vi "Init State Machine.vi"(8 "error in (no error)":errorcluster, 11 "Channel in":refnum<class "Channel.lvclass">) -> (0 "error out":errorcluster, 3 "Channel out":refnum<class "Channel.lvclass">)   [LabVIEW 2018, in "Channel.lvclass"]
doc: "Initialize state machine"
uses:
  Channel.lvclass
  Channel.lvclass/Channel.ctl
  State Machine/CCS_State Machine.lvclass
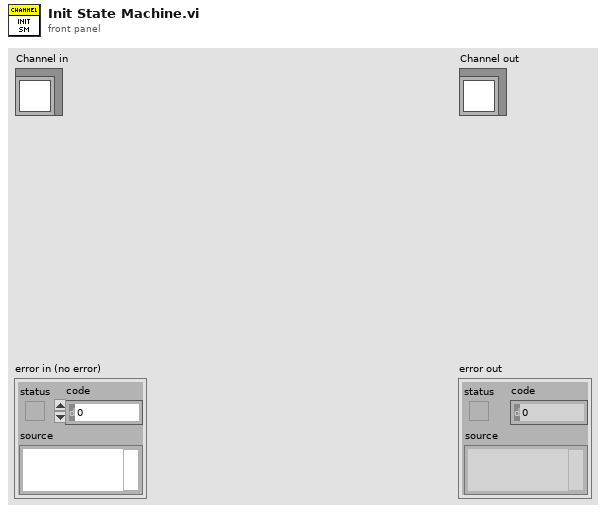
[diagram p1: front panel]
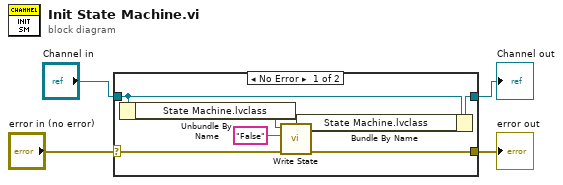
[diagram p0: block diagram]
diagram:
  n1 = case shown="No Error" "error in (no error)" {
    selector: "error in (no error)" -> [w10 w13]
    tunnel: [w11 w13] -> w3
    tunnel: [w8 w12] -> w1
    tunnel: "Channel in" -> [w9 w12]
    frame No Error {
      n2 = Unbundle By Name(w9) -> ("State Machine.lvclass"=w6:refnum<class "CCS_State Machine.lvclass">)
      n3 = call-dynamic "Write State.vi"("error in (no error)"=w10, "State"="False", "State Machine in"=w6) -> ("error out"=w11:errorcluster, "State Machine out"=w5:refnum<class "CCS_State Machine.lvclass">)  [unwired: 7 in]
      n4 = Bundle By Name(cluster=w9, "State Machine.lvclass"=w5) -> (w8:refnum<class "Channel.lvclass">)
    }
    frame Error {
    }
  }
  "error out" <- w3
  "Channel out" <- w1
